vi "Initialize.vi"(8 "error in (no error)":errorcluster, 11 "FlexLogger_gRPCAPI in":refnum<class "FlexLogger_gRPC.lvclass">) -> (0 "error out":errorcluster, 3 "FlexLogger_gRPCAPI out":refnum<class "FlexLogger_gRPC.lvclass">)   [LabVIEW 2020, in "FlexLogger_gRPC.lvlib" / "FlexLogger_gRPC.lvclass"]
doc: "Creates grpc connection with Flexlogger Application running in current system."
uses:
  FlexLogger_gRPC.lvclass
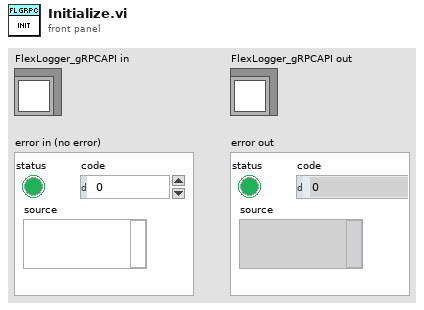
[diagram p1: front panel]
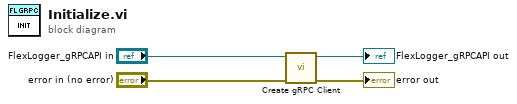
[diagram p0: block diagram]
diagram:
  n1 = call "Create gRPC Client.vi"("error in (no error)"="error in (no error)", "FlexLogger_gRPC in"="FlexLogger_gRPCAPI in") -> ("error out"=→"error out":errorcluster, "FlexLogger_gRPC out"=→"FlexLogger_gRPCAPI out":refnum<class "FlexLogger_gRPC.lvclass">)  [unwired: 8 in]
